vi "SkySparkAcquisitionFGV.vi"(8 "error in (no error)":errorcluster, 10 "FGV_Cluster Input":T1, 11 "Function":T2) -> (0 "error out":errorcluster, 2 "FGV_Cluster Output":T1)   [LabVIEW 2020, in "SkySparkDevice.lvclass"]
uses:
  SkySparkDevice.lvclass
  FGV_TypeDef.ctl
  FGVFunctionTypeDef.ctl
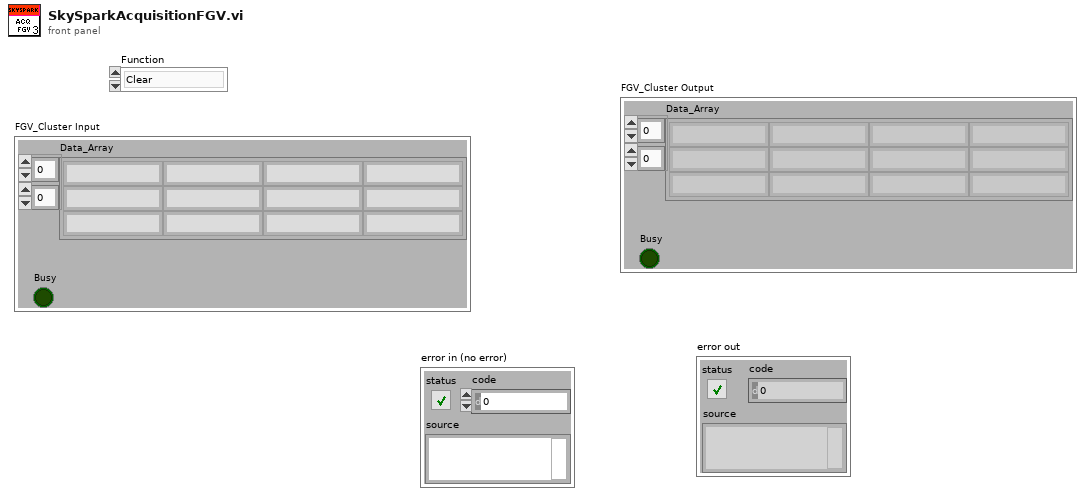
[diagram p1: front panel]
types:
  T1 = typedef "SkySparkDevice.lvclass/FGV_TypeDef.ctl" = cluster{"Data_Array":string[][], "Busy":bool}
  T2 = typedef "SkySparkDevice.lvclass/FGVFunctionTypeDef.ctl" = enum16{"Clear", "Write", "Read"}
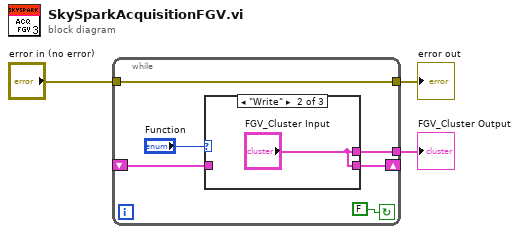
[diagram p0: block diagram]
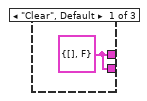
[diagram p2: hidden frame]
diagram:
  n1 = while {
    shift-right: [w7] -> _
    shift-left: _ -> [w6]
    tunnel: [w8] -> w3
    tunnel: "error in (no error)" -> [w4]
    tunnel: [w4] -> w1
    stop <- FALSE continue-if-true
    n2 = case shown="\"Write\"" "Function" {
      tunnel: [w10 "FGV_Cluster Input" w12] -> w8
      tunnel: [w10 "FGV_Cluster Input" w12] -> w7
      tunnel: w6 -> [_ _ w12]
      frame "Clear", Default {
        w10 = T1 {"Data_Array"=[], "Busy"=FALSE} ("FGV_Cluster")
      }
      frame "Write" {
      }
      frame "Read" {
      }
    }
  }
  "FGV_Cluster Output" <- w3
  "error out" <- w1
